vi "File.String Array to CSV.vi"(8 "error in":errorcluster, 9 "2D Array":string[][](array[string]), 10 "Top Row (Header)":string[](array[string]), 11 "File":path=path "C:/Users/eddiek/Documents/01_MTE/Circle Test/Results/ATS_TL/Circle Test Summary Data, 10-06-2017/AB736001B5_CT02_CS01.csv") -> (0 "error out":errorcluster, 3 "Dup File":path)   [LabVIEW 2018]
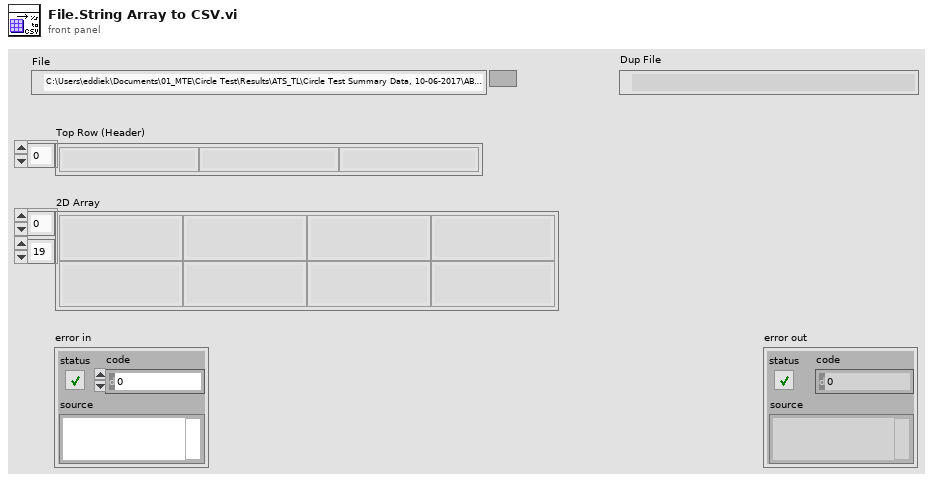
[diagram p1: front panel]
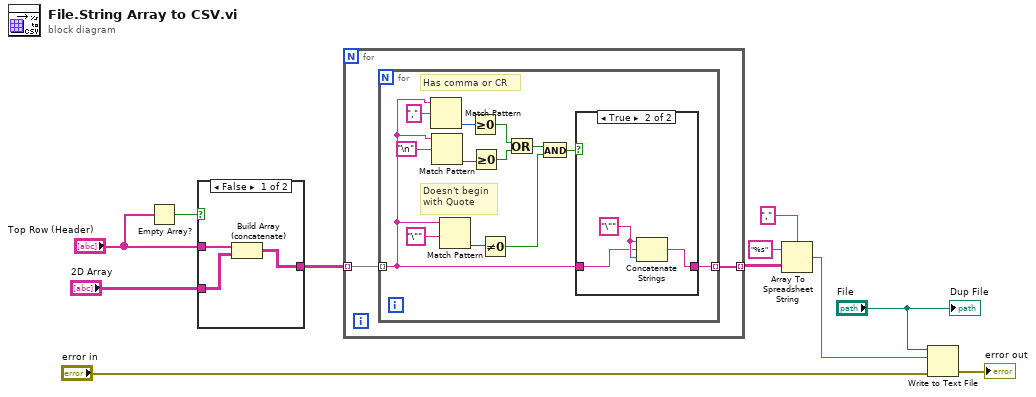
[diagram p0: block diagram]
diagram:
  n1 = Empty Array?(array="Top Row (Header)") -> (empty?=w9:bool)
  n2 = case shown="False" w9 {
    tunnel: "Top Row (Header)" -> [w14 _]
    tunnel: "2D Array" -> [w13 w15]
    tunnel: [w12 w15] -> w5
    frame False {
      n3 = Build Array (concatenate)(w14, w13) -> (w12:string[][])
    }
    frame True {
    }
  }
  n4 = for {
    tunnel: w5 -> [w17] mode=indexing
    tunnel: [w16] -> w4 mode=indexing
    n5 = for {
      tunnel: w17 -> [w18] mode=indexing
      tunnel: [w24] -> w16 mode=indexing
      # "Has comma or CR"
      # "Doesn't begin\nwith Quote"
      n6 = Match Pattern(string=w18, regular expression=",") -> (offset past match=w28:i32)  [unwired: 1 in, 3 out]
      n7 = Match Pattern(string=w18, regular expression="\n") -> (offset past match=w27:i32)  [unwired: 1 in, 3 out]
      n8 = Match Pattern(string=w18, regular expression="\"") -> (offset past match=w23:i32)  [unwired: 1 in, 3 out]
      n9 = Greater Or Equal To 0?(x=w28) -> (x >= 0?=w26:bool)
      n10 = Greater Or Equal To 0?(x=w27) -> (x >= 0?=w25:bool)
      n11 = Not Equal To 0?(x=w23) -> (x != 0?=w19:bool)
      n12 = Or(x=w26, y=w25) -> (x .or. y?=w20:bool)
      n13 = And(x=w20, y=w19) -> (x .and. y?=w21:bool)
      n14 = case shown="True" w21 {
        tunnel: w18 -> [w31 w33]
        tunnel: [w31 w32] -> w24
        frame False {
        }
        frame True {
          w34 = "\""
          n15 = Concatenate Strings(w34, w33, w34) -> (w32:string)
        }
      }
    }
  }
  n16 = Array To Spreadsheet String(delimiter (Tab)=",", array=w4, 3:"%s" ("format string")) -> (spreadsheet string=w1:string)
  n17 = Write to Text File(file (use dialog)="File", text=w1, error in="error in") -> (error out=→"error out":errorcluster)  [unwired: 1 in, 2 out]
  "Dup File" <- "File"
